vi "Write Request.vi"(8 "error in (no error)":errorcluster, 9 "params":string[](array[string]), 10 "method":string, 11 "JSON RPC in":refnum<class "JSON RPC.lvclass">) -> (0 "error out":errorcluster, 2 "JSON string":string, 3 "JSON RPC out":refnum<class "JSON RPC.lvclass">)   [LabVIEW 2016, in "JSON RPC.lvclass"]
uses:
  JSON RPC.lvclass
  JSON RPC.lvclass/JSON RPC.ctl
  <vilib>/httpClient/POSTBuffer.vi
  <vilib>/httpClient/LabVIEWHTTPClient.lvlib
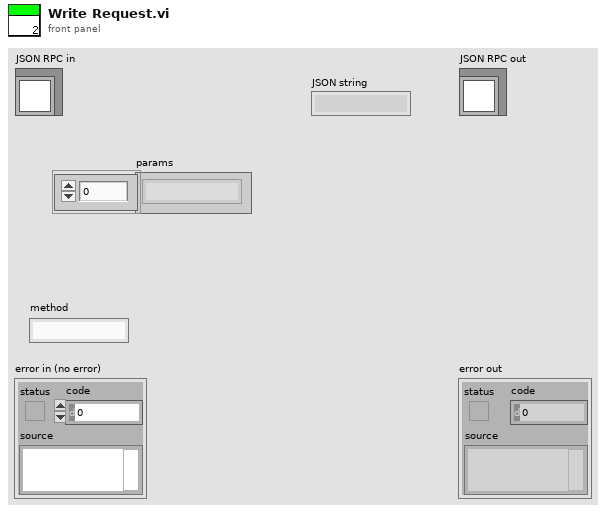
[diagram p1: front panel]
types:
  T1 = cluster{"params[0]":string, "params[1]":string, "params[2]":string, "params[3]":string, "params[4]":string, "params[5]":string, "params[6]":string, "params[7]":string, "params[8]":string}
  T2 = cluster{"id":string, "jsonrpc":string, "method":string, "params":string[]}
  T3 = cluster{"id":string, "jsonrpc":string, "method":string}
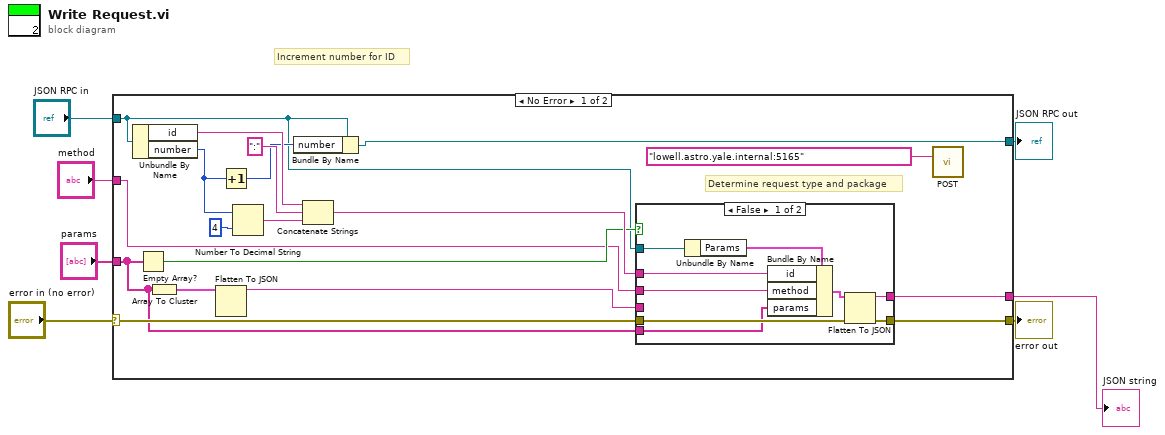
[diagram p0: block diagram]
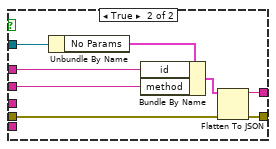
[diagram p2: hidden frame]
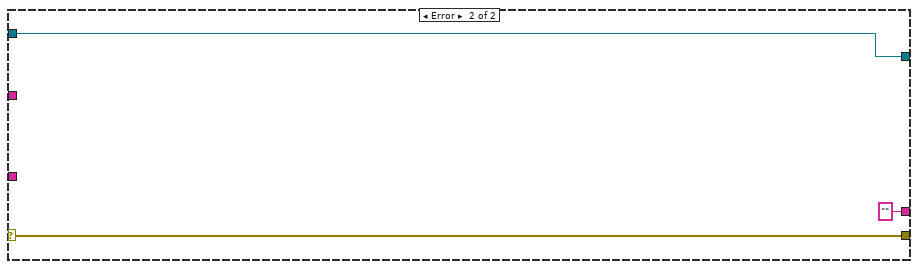
[diagram p3: hidden frame]
diagram:
  # "Increment number for ID"
  n1 = case shown="No Error" "error in (no error)" {
    selector: "error in (no error)" -> [w11 w45]
    tunnel: [w10 w45] -> w6
    tunnel: "JSON RPC in" -> [w16 w44]
    tunnel: "method" -> [w17 _]
    tunnel: "params" -> [w8 _]
    tunnel: [w13 w44] -> w2
    tunnel: [w9 "" ("JSON string")] -> w1
    frame No Error {
      # "Determine request type and package"
      n2 = Unbundle By Name(w16) -> ("id"=w24:string, "number"=w20:i32)
      n3 = Empty Array?(array=w8) -> (empty?=w18:bool)
      n4 = Array To Cluster(array=w8) -> (cluster=w14:T1)
      n5 = Flatten To JSON(anything=w14) -> (JSON string=w15:string)  [unwired: 2 in, 1 out]
      n6 = Increment(x=w20) -> (x+1=w21:i32)
      n7 = Number To Decimal String(number=w20, width (-)=i16 4) -> (decimal integer string=w23:string)
      n8 = Bundle By Name(cluster=w16, "number"=w21) -> (w13:refnum<class "JSON RPC.lvclass">)
      n9 = Concatenate Strings(w24, ":" ("string"), w23) -> (w19:string)
      n10 = case shown="False" w18 {
        tunnel: w19 -> [w34 w40]
        tunnel: w17 -> [w33 w39]
        tunnel: w16 -> [w32 w42]
        tunnel: w15 -> [_ _]
        tunnel: [w29 w37] -> w9
        tunnel: w11 -> [w28 w36]
        tunnel: [w27 w35] -> w10
        tunnel: w8 -> [w26 _]
        frame False {
          n11 = Unbundle By Name(w32) -> ("Params"=w31:T2)
          n12 = Bundle By Name(cluster=w31, "id"=w34, "method"=w33, "params"=w26) -> (w30:T2)
          n13 = Flatten To JSON(anything=w30, error in (no error)=w28) -> (JSON string=w29:string, 11:w27:errorcluster)  [unwired: 1 in]
        }
        frame True {
          n14 = Unbundle By Name(w42) -> ("No Params"=w41:T3)
          n15 = Bundle By Name(cluster=w41, "id"=w40, "method"=w39) -> (w38:T3)
          n16 = Flatten To JSON(anything=w38, error in (no error)=w36) -> (JSON string=w37:string, 11:w35:errorcluster)  [unwired: 1 in]
        }
      }
      n17 = call-poly <vilib>:"POST.vi"("url"="lowell.astro.yale.internal:5165") -> ()  [unwired: 11 in, 4 out]
    }
    frame Error {
    }
  }
  "error out" <- w6
  "JSON RPC out" <- w2
  "JSON string" <- w1
